vi "CONEX-LDS Set Laser Power Enable v2.vi"(7 "Laser Enable (F)":bool, 9 "Connection Cluster in":T1) -> (3 "Connection Cluster out":T1)   [LabVIEW 2010]
doc: "Laser Enable State to Enabled or Disabled.\n\nInput: Laser Enable (F)\nT - Enabled - Laser On.\nF - Disabled - Laser Off."
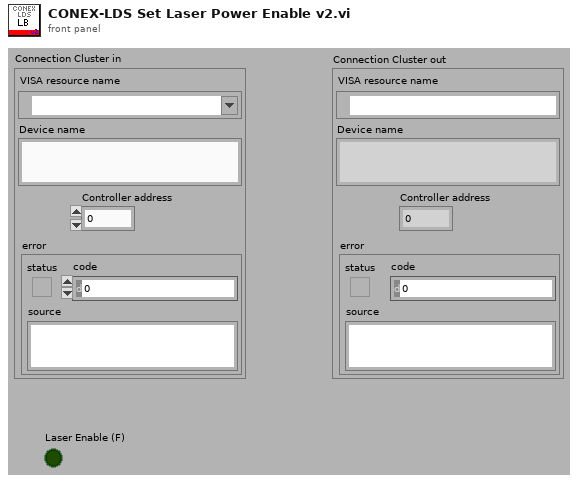
[diagram p1: front panel]
types:
  T1 = cluster{"VISA resource name":refnum<visa-resource-name>, "Device name":string, "Controller address":i32, "error":errorcluster}
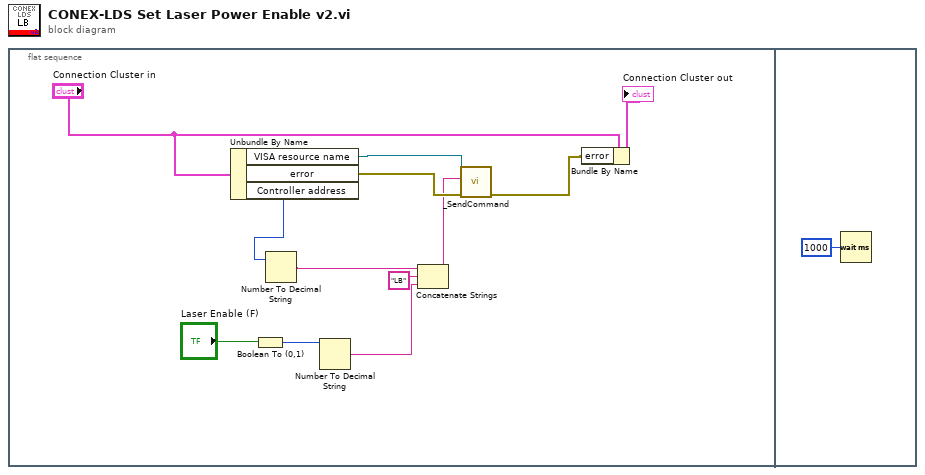
[diagram p0: block diagram]
diagram:
  n1 = flat-sequence {
    frame #0 {
      n2 = Unbundle By Name("Connection Cluster in") -> ("VISA resource name"=w7:refnum<visa-resource-name>, "error"=w5:errorcluster, "Controller address"=w4:i32)
      n3 = Boolean To (0,1)(Boolean="Laser Enable (F)") -> (0, 1=w9:i16)
      n4 = Number To Decimal String(number=w4) -> (decimal integer string=w12:string)  [unwired: 1 out]
      n5 = Number To Decimal String(number=w9) -> (decimal integer string=w8:string)  [unwired: 1 out]
      n6 = Concatenate Strings(w12, "LB" ("strCommand"), w8) -> (w1:string)
      n7 = call <userlib>:"_SendCommand.vi"("error in"=w5, "Command"=w1, "Instrument Channel"=w7) -> ("error out"=w6:errorcluster)  [unwired: 7 in, 1 out]
      n8 = Bundle By Name(cluster="Connection Cluster in", "error"=w6) -> (→"Connection Cluster out":T1)
    }
    frame #1 {
      n9 = Wait (ms)(milliseconds to wait=u32 1000 ("attente (ms)")) -> ()  [unwired: 1 out]
    }
  }
